vi "Logging.vi"(4 "Log Stream":T1, 11 "Log Msg":T2) -> (6 "UI Msg":T2)   [LabVIEW 2019, in "Logging.lvlib"]
doc: "The message loop subVI to handle messages pertaining to logging data."
uses:
  Logging.lvlib
  <extravilib>/ChannelInstances/Messenger-t'Message Queue.lvlib-Message Cluster.ctl'/))Channel.ctl
  support/Message Queue/Message Cluster.ctl
  <extravilib>/ChannelInstances/Stream-var/)Channel.ctl
  Logging Conf.ctl
  Logging State.ctl
  HeatFlow/HeatFlow Res Cfg.ctl
  <vilib>/Utility/error.llb/Error Cluster From Error Code.vi
  <vilib>/ErrorRing/Error Ring.xnode
  support/Message Queue/Message Queue.lvlib
  <extravilib>/ChannelInstances/Messenger-t'Message Queue.lvlib-Message Cluster.ctl'.lvlib
  <extravilib>/ChannelInstances/Stream-var.lvlib
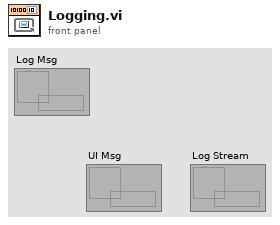
[diagram p1: front panel]
types:
  T1 = typedef "Stream-var.lvlib/)Channel.ctl" = refnum<queue>
  T2 = typedef "Messenger-t'Message Queue.lvlib-Message Cluster.ctl'.lvlib/))Channel.ctl" = refnum<queue>
  T3 = typedef "Logging.lvlib/HeatFlow Res Cfg.ctl" = cluster{"Heater Temp":cluster{"On":bool, "Min Val":dbl, "Max Val":dbl, "Units":string}, "Tube Temp":cluster{"On":bool, "Min Val":dbl, "Max Val":dbl, "Units":string}, "Hot Heater Power":cluster{"On":bool, "Min Val":dbl, "Max Val":dbl, "Units":string}, "TEG Power":cluster{"On":bool, "Min Val":dbl, "Max Val":dbl, "Units":string}, "Details":bool, "Heater dU":cluster{"Min Val":dbl, "Max Val":dbl, "Units":string}, "I Res dU":cluster{"Min Val":dbl, "Max Val":dbl, "Units":string}}
  T4 = typedef "Logging.lvlib/Logging State.ctl" = enum16{"Idle", "Logging"}
  T5 = typedef "Logging.lvlib/Logging Conf.ctl" = cluster{"Log File Base Path":path, "TDMS File Reference":refnum<k34>}
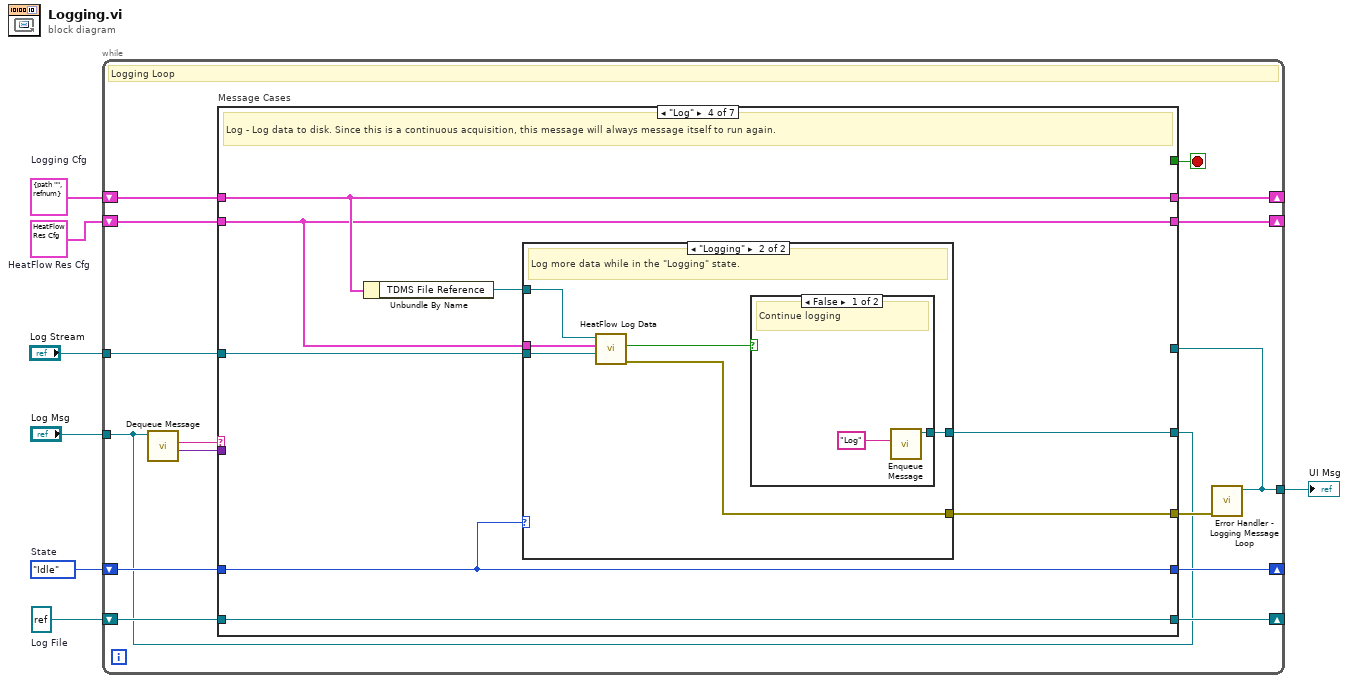
[diagram p0: block diagram]
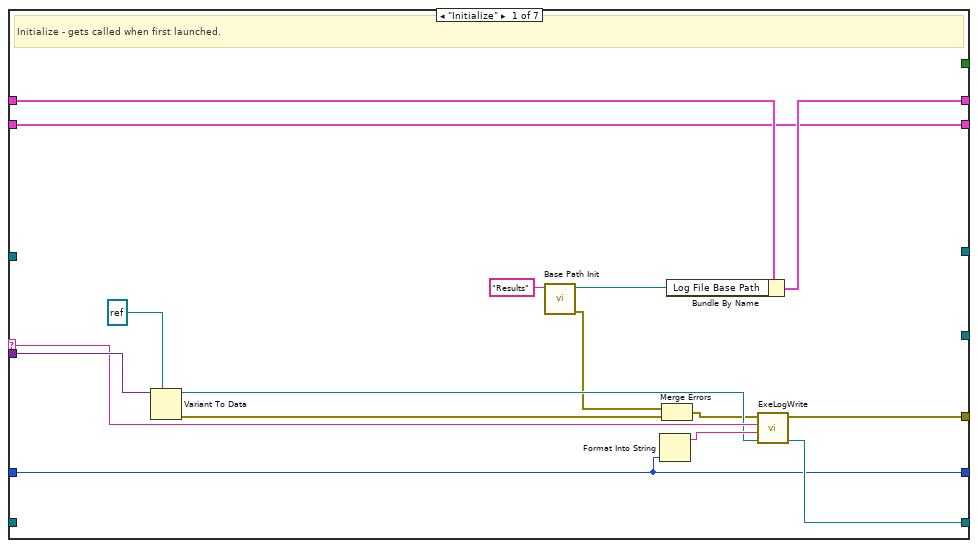
[diagram p2: hidden frame]
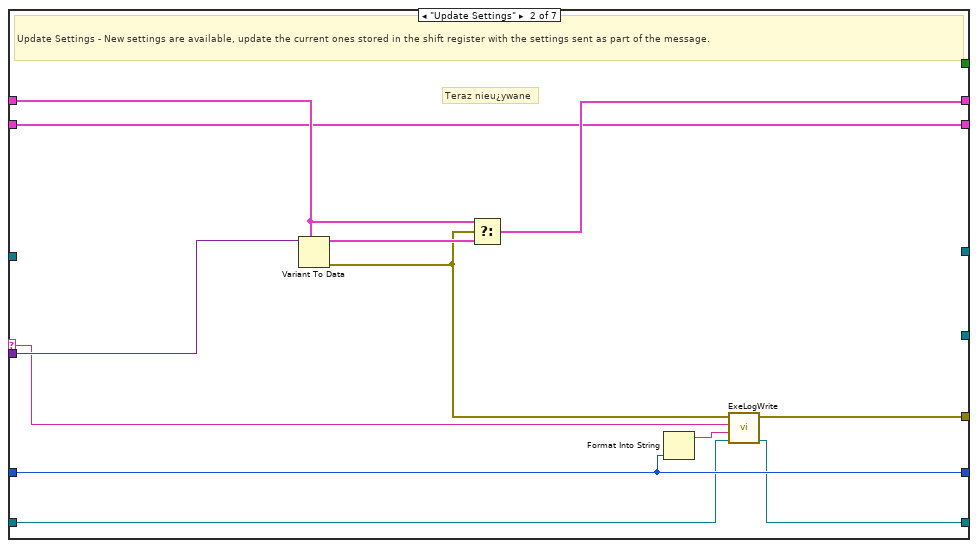
[diagram p3: hidden frame]
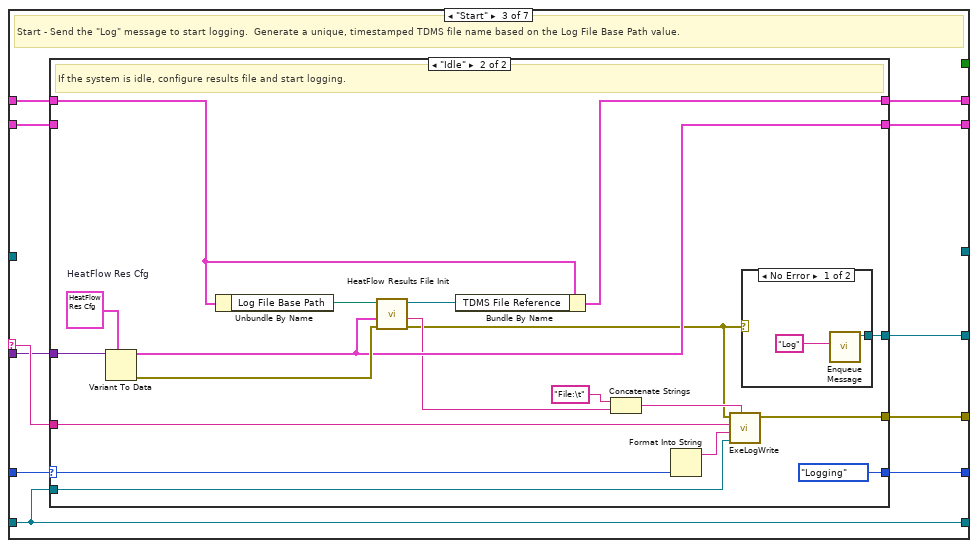
[diagram p4: hidden frame]
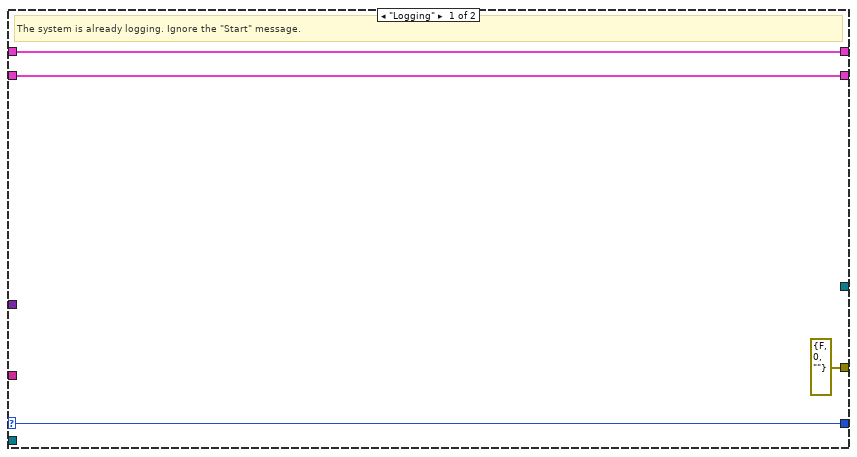
[diagram p5: hidden frame]
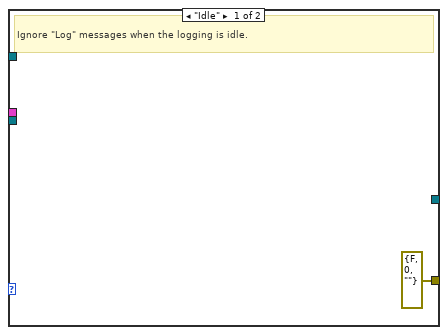
[diagram p7: hidden frame]
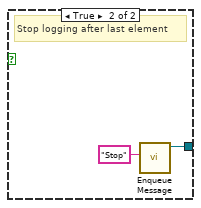
[diagram p8: hidden frame]
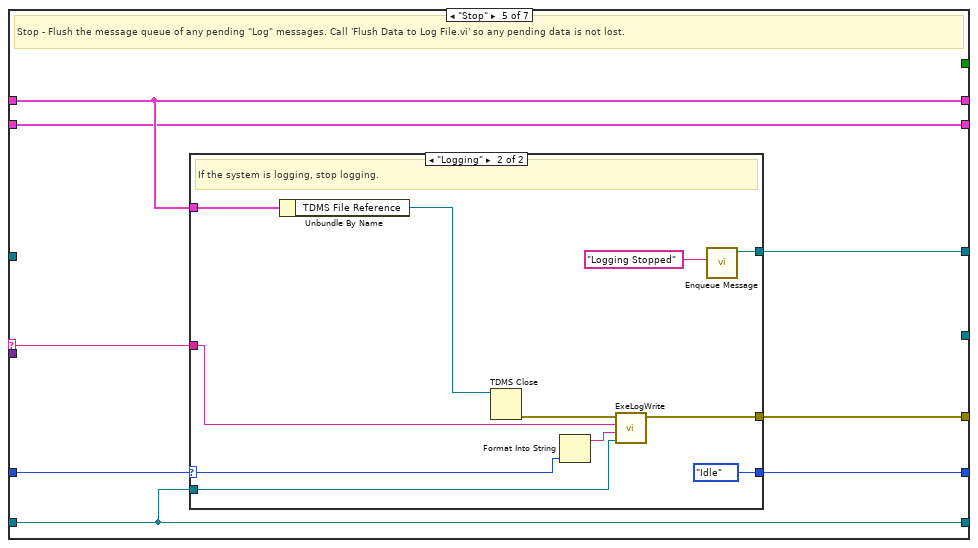
[diagram p9: hidden frame]
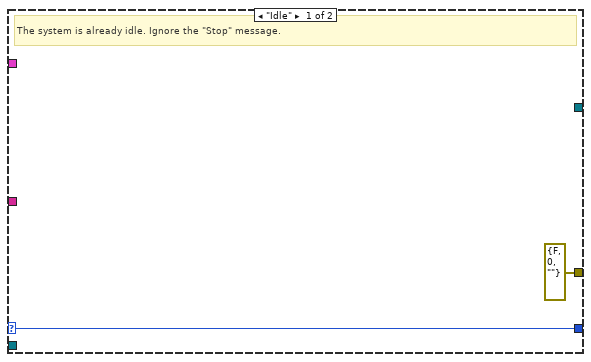
[diagram p10: hidden frame]
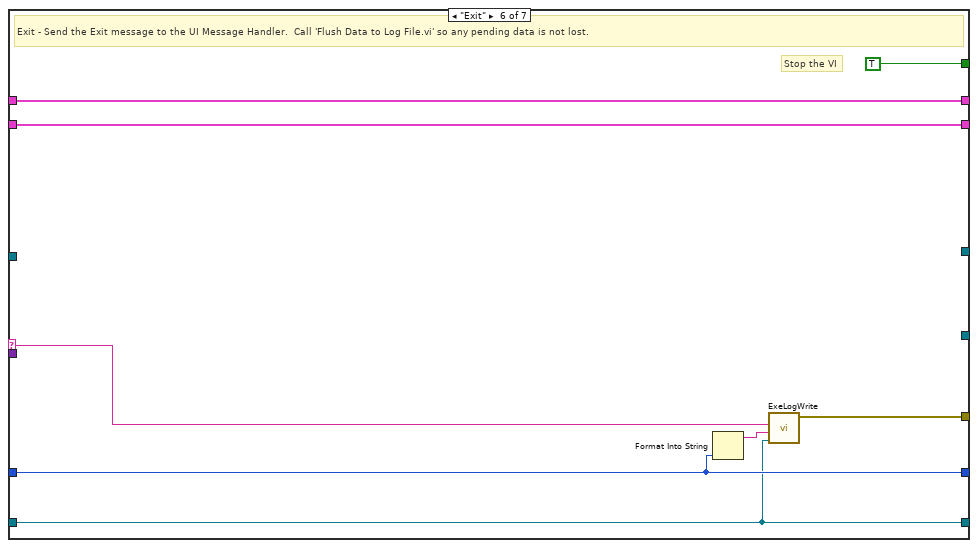
[diagram p11: hidden frame]
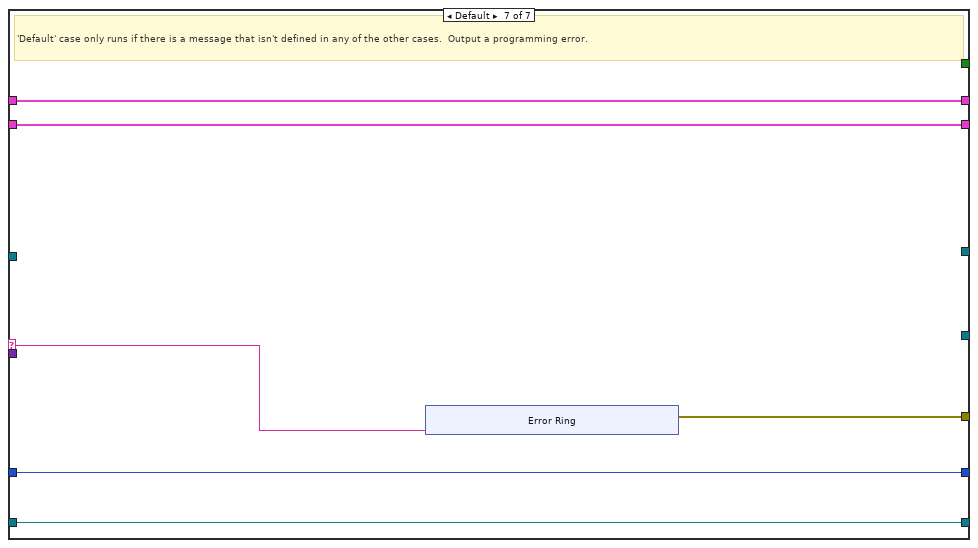
[diagram p12: hidden frame]
diagram:
  w1 = T3 {"Heater Temp"={"On"=FALSE, "Min Val"=0.0, "Max Val"=0.0, "Units"=""}, "Tube Temp"={"On"=FALSE, "Min Val"=0.0, "Max Val"=0.0, "Units"=""}, "Hot Heater Power"={"On"=FALSE, "Min Val"=0.0, "Max Val"=0.0, "Units"=""}, "TEG Power"={"On"=FALSE, "Min Val"=0.0, "Max Val"=0.0, "Units"=""}, "Details"=FALSE, "Heater dU"={"Min Val"=0.0, "Max Val"=0.0, "Units"=""}, "I Res dU"={"Min Val"=0.0, "Max Val"=0.0, "Units"=""}}  # HeatFlow Res Cfg
  w3 = refnum<file> refnum  # Log File
  w4 = Logging_State."Idle"  # State
  w5 = T5 {"Log File Base Path"=path "", "TDMS File Reference"=refnum}  # Logging Cfg
  n1 = while {
    shift-right: [w21] -> _
    shift-left: w5 -> [w22]
    shift-right: [w19] -> _
    shift-left: w4 -> [w20]
    tunnel: "Log Msg" -> [w10]
    tunnel: [w14] -> w7
    tunnel: "Log Stream" -> [w15]
    shift-right: [w11] -> _
    shift-left: w3 -> [w12]
    shift-right: [w8] -> _
    shift-left: w1 -> [w9]
    stop <- w13 stop-if-true
    # "Logging Loop"
    n2 = call "Dequeue Message.vi"("channel"=w10) -> ("message data"=w16:variant, "message"=w17:string)  [unwired: 8 in, 1 out]
    n3 = case "Message Cases" shown="\"Log\"" w17 {
      selector: w17 -> [w36 w43 w54 _ w107 w128 w137]
      tunnel: [w34 w46 w61 w94 w109 w132 w138] -> w18
      tunnel: w22 -> [w31 w50 w60 w90 w110 w134 w140]
      tunnel: [w30 w48 w59 w90 w110 w134 w140] -> w21
      tunnel: w20 -> [w29 w42 w58 w88 w113 w130 w139]
      tunnel: [w29 w42 w57 w88 w112 w130 w139] -> w19
      tunnel: w16 -> [w38 w47 w53 _ _ _ _]
      tunnel: [_ _ w56 w93 _ _ _] -> w10
      tunnel: w15 -> [_ _ _ w92 _ _ _]
      tunnel: [_ _ _ _ w111 _ _] -> w14
      tunnel: [_ _ _ _ _ TRUE _] -> w13
      tunnel: w12 -> [_ w41 w55 w91 w108 w129 w136]
      tunnel: [w33 w40 w55 w91 w108 w129 w136] -> w11
      tunnel: w9 -> [w23 w39 w52 w87 w106 w127 w135]
      tunnel: [w23 w39 w51 w87 w106 w127 w135] -> w8
      frame "Initialize" {
        # "Initialize - gets called when first launched."
        n4 = Variant To Data(type=refnum<file> refnum ("refnum out"), Variant=w38) -> (data=w28:refnum<file>, error out=w27:errorcluster)  [unwired: 1 in]
        n5 = call "Base Path Init.vi"("Folder name"="Results" ("name or relative path")) -> ("error out"=w24:errorcluster, "Folder Path"=w25:path)  [unwired: 9 in]
        n6 = Format Into String(w29) -> (resulting string=w35:string)  [unwired: 3 in, 1 out]
        n7 = Merge Errors(w24, w27) -> (w26:errorcluster)
        n8 = Bundle By Name(cluster=w31, "Log File Base Path"=w25) -> (w30:T5)
        n9 = call "ExeLogWrite.vi"("refnum in"=w28, "State"=w35, "Message"=w36, "error in"=w26) -> ("refnum out"=w33:refnum<file>, "error out"=w34:errorcluster)  [unwired: 6 in]
      }
      frame "Update Settings" {
        # "Teraz nieu¿ywane"
        # "Update Settings - New settings are available, update the current ones stored in the shift register with the settings sent as part of the message."
        n10 = Variant To Data(type=w50, Variant=w47) -> (data=w49:T5, error out=w45:errorcluster)  [unwired: 1 in]
        n11 = Select(t=w50, s=w45, f=w49) -> (s? t:f=w48:T5)
        n12 = Format Into String(w42) -> (resulting string=w44:string)  [unwired: 3 in, 1 out]
        n13 = call "ExeLogWrite.vi"("refnum in"=w41, "State"=w44, "Message"=w43, "error in"=w45) -> ("refnum out"=w40:refnum<file>, "error out"=w46:errorcluster)  [unwired: 6 in]
      }
      frame "Start" {
        # "Start - Send the \"Log\" message to start logging.  Generate a unique, timestamped TDMS file name based on the Log File Base Path value."
        n14 = case shown="\"Idle\"" w58 {
          selector: w58 -> [w64 w78]
          tunnel: [errorcluster {"status"=FALSE, "code"=0, "source"=""} ("error out") w80] -> w61
          tunnel: w60 -> [w65 w82]
          tunnel: [w65 w84] -> w59
          tunnel: [w64 Logging_State."Logging" ("State")] -> w57
          tunnel: [_ w81] -> w56
          tunnel: w55 -> [_ w79]
          tunnel: w54 -> [_ w76]
          tunnel: w53 -> [_ w73]
          tunnel: w52 -> [w62 _]
          tunnel: [w62 w69] -> w51
          frame "Logging" {
            # "The system is already logging. Ignore the \"Start\" message."
          }
          frame "Idle" {
            w66 = T3 {"Heater Temp"={"On"=FALSE, "Min Val"=0.0, "Max Val"=0.0, "Units"=""}, "Tube Temp"={"On"=FALSE, "Min Val"=0.0, "Max Val"=0.0, "Units"=""}, "Hot Heater Power"={"On"=FALSE, "Min Val"=0.0, "Max Val"=0.0, "Units"=""}, "TEG Power"={"On"=FALSE, "Min Val"=0.0, "Max Val"=0.0, "Units"=""}, "Details"=FALSE, "Heater dU"={"Min Val"=0.0, "Max Val"=0.0, "Units"=""}, "I Res dU"={"Min Val"=0.0, "Max Val"=0.0, "Units"=""}}  # HeatFlow Res Cfg
            # "If the system is idle, configure results file and start logging."
            n15 = Variant To Data(type=w66, Variant=w73) -> (data=w69:T3, error out=w72:errorcluster)  [unwired: 1 in]
            n16 = Unbundle By Name(w82) -> ("Log File Base Path"=w71:path)
            n17 = call "HeatFlow Results File Init.vi"("error in"=w72, "HeatFlow Res Cfg"=w69, "Log File Base Path"=w71) -> ("error out"=w67:errorcluster, "Log File Name"=w68:string, "Refnum out"=w70:refnum<k34>)  [unwired: 6 in]
            n18 = Bundle By Name(cluster=w82, "TDMS File Reference"=w70) -> (w84:T5)
            n19 = Concatenate Strings("File:\t" ("string"), w68) -> (w74:string)
            n20 = Format Into String(w78) -> (resulting string=w77:string)  [unwired: 3 in, 1 out]
            n21 = call "ExeLogWrite.vi"("Extra"=w74, "refnum in"=w79, "State"=w77, "Message"=w76, "error in"=w67) -> ("error out"=w80:errorcluster)  [unwired: 5 in, 1 out]
            n22 = case shown="No Error" w67 {
              tunnel: [w85 _] -> w81
              frame No Error {
                n23 = call "Enqueue Message.vi"("message"="Log" ("Message")) -> ("channel"=w85:T2)  [unwired: 10 in]
              }
              frame Error {
              }
            }
          }
        }
      }
      frame "Log" {
        # "Log - Log data to disk. Since this is a continuous acquisition, this message will always message itself to run again."
        n24 = Unbundle By Name(w90) -> ("TDMS File Reference"=w89:refnum<k34>)
        n25 = case shown="\"Logging\"" w88 {
          tunnel: [errorcluster {"status"=FALSE, "code"=0, "source"=""} ("error out") w97] -> w94
          tunnel: [_ w101] -> w93
          tunnel: w92 -> [_ w100]
          tunnel: w89 -> [_ w98]
          tunnel: w87 -> [_ w96]
          frame "Idle" {
            # "Ignore \"Log\" messages when the logging is idle."
          }
          frame "Logging" {
            # "Log more data while in the \"Logging\" state."
            n26 = call "HeatFlow Log Data.vi"("Log Stream"=w100, "HeatFlow Res Cfg"=w96, "tdms file"=w98) -> ("error out"=w97:errorcluster, "Acquisition Stopped?"=w99:bool)  [unwired: 7 in]
            n27 = case shown="False" w99 {
              tunnel: [w102 w105] -> w101
              frame False {
                # "Continue logging"
                n28 = call "Enqueue Message.vi"("message"="Log" ("Message")) -> ("channel"=w102:T2)  [unwired: 10 in]
              }
              frame True {
                # "Stop logging after last element"
                n29 = call "Enqueue Message.vi"("message"="Stop") -> ("channel"=w105:T2)  [unwired: 10 in]
              }
            }
          }
        }
      }
      frame "Stop" {
        # "Stop - Flush the message queue of any pending \"Log\" messages. Call 'Flush Data to Log File.vi' so any pending data is not lost."
        n30 = case shown="\"Logging\"" w113 {
          selector: w113 -> [w115 w119]
          tunnel: w110 -> [_ w123]
          tunnel: [w115 Logging_State."Idle" ("State")] -> w112
          tunnel: [errorcluster {"status"=FALSE, "code"=0, "source"=""} ("error out") w121] -> w109
          tunnel: [_ w125] -> w111
          tunnel: w108 -> [_ w117]
          tunnel: w107 -> [_ w116]
          frame "Idle" {
            # "The system is already idle. Ignore the \"Stop\" message."
          }
          frame "Logging" {
            # "If the system is logging, stop logging."
            n31 = Unbundle By Name(w123) -> ("TDMS File Reference"=w122:refnum<k34>)
            n32 = TDMS Close(11:w122) -> (0:w120:errorcluster)  [unwired: 1 in, 1 out]
            n33 = Format Into String(w119) -> (resulting string=w118:string)  [unwired: 3 in, 1 out]
            n34 = call "ExeLogWrite.vi"("refnum in"=w117, "State"=w118, "Message"=w116, "error in"=w120) -> ("error out"=w121:errorcluster)  [unwired: 6 in, 1 out]
            n35 = call "Enqueue Message.vi"("message"="Logging Stopped") -> ("channel"=w125:T2)  [unwired: 10 in]
          }
        }
      }
      frame "Exit" {
        # "Stop the VI"
        # "Exit - Send the Exit message to the UI Message Handler.  Call 'Flush Data to Log File.vi' so any pending data is not lost."
        n36 = Format Into String(w130) -> (resulting string=w131:string)  [unwired: 3 in, 1 out]
        n37 = call "ExeLogWrite.vi"("refnum in"=w129, "State"=w131, "Message"=w128) -> ("error out"=w132:errorcluster)  [unwired: 7 in, 1 out]
      }
      frame Default {
        # "'Default' case only runs if there is a message that isn't defined in any of the other cases.  Output a programming error."
        n38 = xnode "Error Ring"("parameter 0"=w137) -> ("error out"=w138:errorcluster)
      }
    }
    n39 = call "Error Handler - Logging Message Loop.vi"("UI Channel"=w14, "error in (no error)"=w18) -> ()  [unwired: 9 in, 1 out]
  }
  "UI Msg" <- w7
